vi "Set Defaults from Strings.vi"(8 "error in (no error)":errorcluster, 10 "Default Strings":string[](array[string]), 11 "Group in":refnum<class "Group DBL.lvclass">) -> (0 "error out":errorcluster, 3 "Group out":refnum<class "Group DBL.lvclass">)   [LabVIEW 2020, in "Vecto.lvlib" / "Group DBL.lvclass"]
uses:
  Group DBL.lvclass
  Group DBL.lvclass/Group DBL.ctl
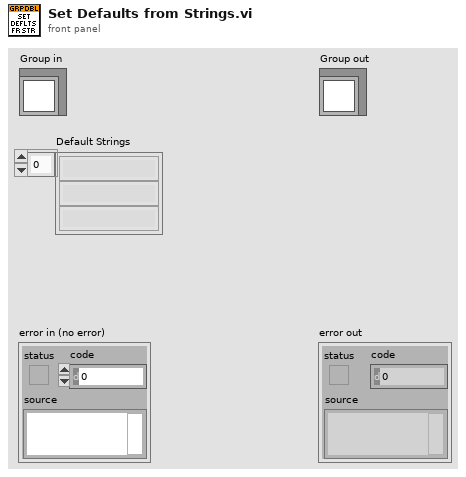
[diagram p1: front panel]
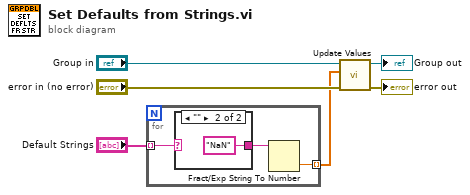
[diagram p0: block diagram]
diagram:
  n1 = for {
    tunnel: "Default Strings" -> [w9] mode=indexing
    tunnel: [w7] -> w1 mode=indexing
    n2 = case shown="\"\"" w9 {
      selector: w9 -> [w10 _]
      tunnel: [w10 "NaN"] -> w8
      frame Default {
      }
      frame "" {
      }
    }
    n3 = Fract/Exp String To Number(string=w8) -> (number=w7:dbl)  [unwired: 3 in, 1 out]
  }
  n4 = call "Update Values.vi"("error in (no error)"="error in (no error)", "Values"=w1, "Group in"="Group in") -> ("error out"=→"error out":errorcluster, "Group out"=→"Group out":refnum<class "Group DBL.lvclass">)  [unwired: 7 in]
